vi "IPS Set Control.vi"(4 "Error In":errorcluster, 6 "Control":T1, 7 "VISA resource name":refnum<visa-resource-name>="GPIB1::24::INSTR") -> (0 "Error Out":errorcluster, 1 "Response":string="C\r", 3 "VISA resource name":refnum<visa-resource-name>="GPIB1::25::INSTR")   [LabVIEW 2016, in "IPS-120.lvlib"]
uses:
  IPS-120.lvlib
  Typedefs/Set Control - Enum.ctl
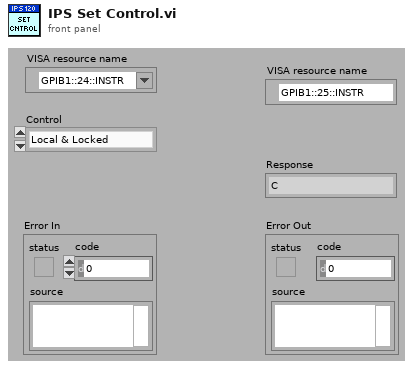
[diagram p1: front panel]
types:
  T1 = typedef "IPS-120.lvlib/Set Control - Enum.ctl" = enum16{"Local & Locked", "Remote & Locked", "Local & Unlocked", "Remote & Unlocked"}
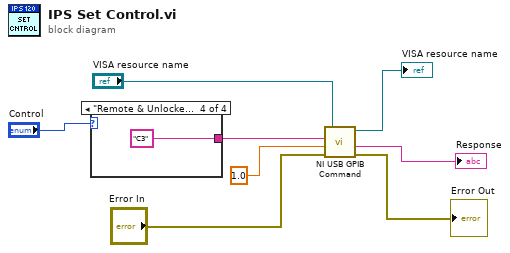
[diagram p0: block diagram]
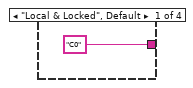
[diagram p2: hidden frame]
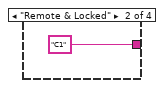
[diagram p3: hidden frame]
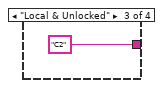
[diagram p4: hidden frame]
diagram:
  n1 = case shown="\"Remote & Unlocked\"" "Control" {
    tunnel: ["C0" ("String to Send") "C1" ("String to Send") "C2" ("String to Send") "C3" ("String to Send")] -> w6
    frame "Local & Locked", Default {
    }
    frame "Remote & Locked" {
    }
    frame "Local & Unlocked" {
    }
    frame "Remote & Unlocked" {
    }
  }
  n2 = call "NI USB GPIB Command.vi"("Error In"="Error In", "Wait for instrument to respond (s)"=1.0, "String to Send"=w6, "VISA resource name"="VISA resource name") -> ("Error Out"=→"Error Out":errorcluster, "Return String from Device (Not all commands return a String)"=→"Response":string, "VISA resource name out"=→"VISA resource name":refnum<visa-resource-name>)  [unwired: 1 out]
